vi "Flatten Jacobian.vi"(10 "Gradient In":T1[](array[typedef]), 11 "Jacobian":T1[][](array[typedef])) -> (3 "Gradient Out":T1[](array[typedef]))   [LabVIEW 2011, in "Super Simple Neural Network.lvlib"]
uses:
  Super Simple Neural Network.lvlib
  Types/2D Array.ctl
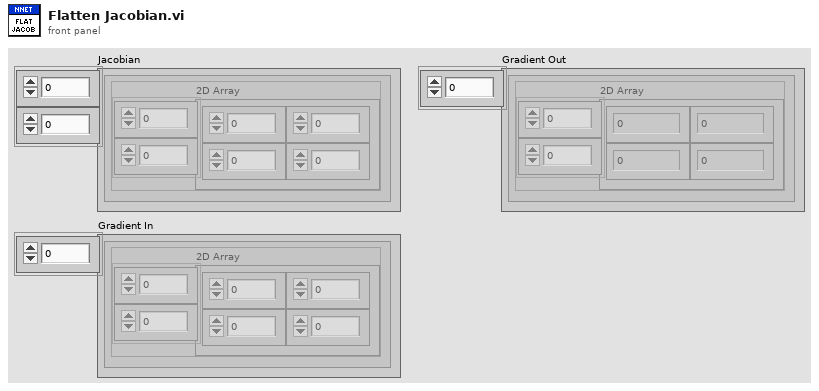
[diagram p1: front panel]
types:
  T1 = typedef "Super Simple Neural Network.lvlib/2D Array.ctl" = cluster{"2D Array":dbl[][]}
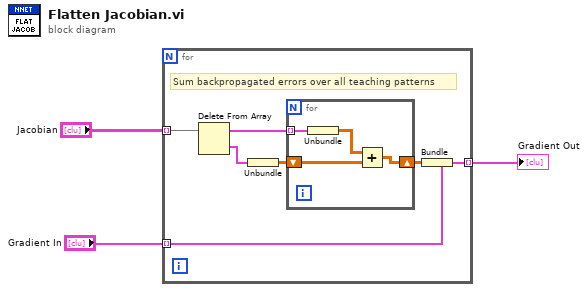
[diagram p0: block diagram]
diagram:
  n1 = for {
    tunnel: "Jacobian" -> [w7] mode=indexing
    tunnel: [w6] -> w1 mode=indexing
    tunnel: "Gradient In" -> [w4] mode=indexing
    # "Sum backpropagated errors over all teaching patterns"
    n2 = Delete From Array(array=w7) -> (deleted portion=w10:T1, array with subset deleted=w8:T1[])  [unwired: 2 in]
    n3 = Unbundle(w10) -> ("2D Array"=w9:dbl[][])
    n4 = for {
      tunnel: w8 -> [w14] mode=indexing
      shift-right: [w11] -> w5
      shift-left: w9 -> [w13]
      n5 = Unbundle(w14) -> ("2D Array"=w12:dbl[][])
      n6 = Add(x=w12, y=w13) -> (x+y=w11:dbl[][])
    }
    n7 = Bundle(cluster=w4, "2D Array"=w5) -> (w6:T1)
  }
  "Gradient Out" <- w1
